vi "Loop count.vi"() -> ()   [LabVIEW 2018]
panel:
  out "Loop count":dbl
  in  "Power":bool
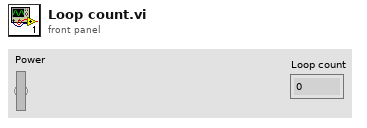
[diagram p1: front panel]
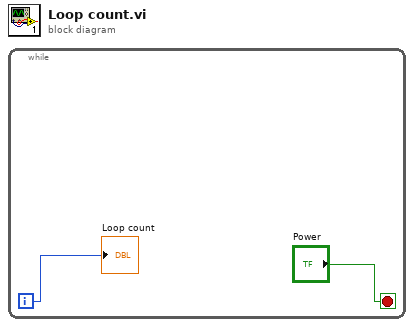
[diagram p0: block diagram]
diagram:
  n1 = while {
    i -> [w1]
    stop <- "Power" stop-if-true
    "Loop count" <- w1
  }
